vi "LJM_eAddresses Example.vi"() -> (0 "error out":errorcluster)   [LabVIEW 2020]
panel:
  in  "Write/Read":i32[](array[ring])=[1, 1, 0, 0, 0, 0] items=["Read", "Write"]
  out "Values Out":dbl[][](array[numeric]) format="%.2f"
  in  "Values In":dbl[][](array[numeric])=[[2.5], [12345.0], [0.0], [0.0], [0.0], [0.0]] format="%.2f"
  in  "NumValues":u16[](array[numeric])=[1, 1, 1, 1, 1, 1]
  in  "Types":u8[](array[numeric])=[3, 0, 0, 1, 3, 3]
  in  "Addresses":u16[](array[numeric])=[1000, 55110, 55110, 60028, 60000, 60004]
  out "Error String":string
  out "ConnectionType Out":i32
  out "DeviceType Out":i32
  in  "Identifier":string="LJM_idANY"
  in  "ConnectionType":string="LJM_ctANY"
  in  "DeviceType":string="LJM_dtANY"
  out "ErrorAddress":i32
  # "Common Registers:\nAddress, Name, Type, Read/Write\n0, AIN0, 3, RO\n2, AIN1, 3, RO\n1000, DAC0, 3, RW\n1002, DAC1, 3, RW\n2000, FIO0, 0, RW\n2001, FIO1, 0, RW\n55110, TEST_UINT16, 0, RW\n60000, PRODUCT_ID, 3, RO\n60004, FIRMWARE_VERSION, 3, RO\n60028, SERIAL_NUMBER, 1, RO\n\nTypes: 0=UINT16, 1=UINT32, 2=INT32, 3=FLOAT32"
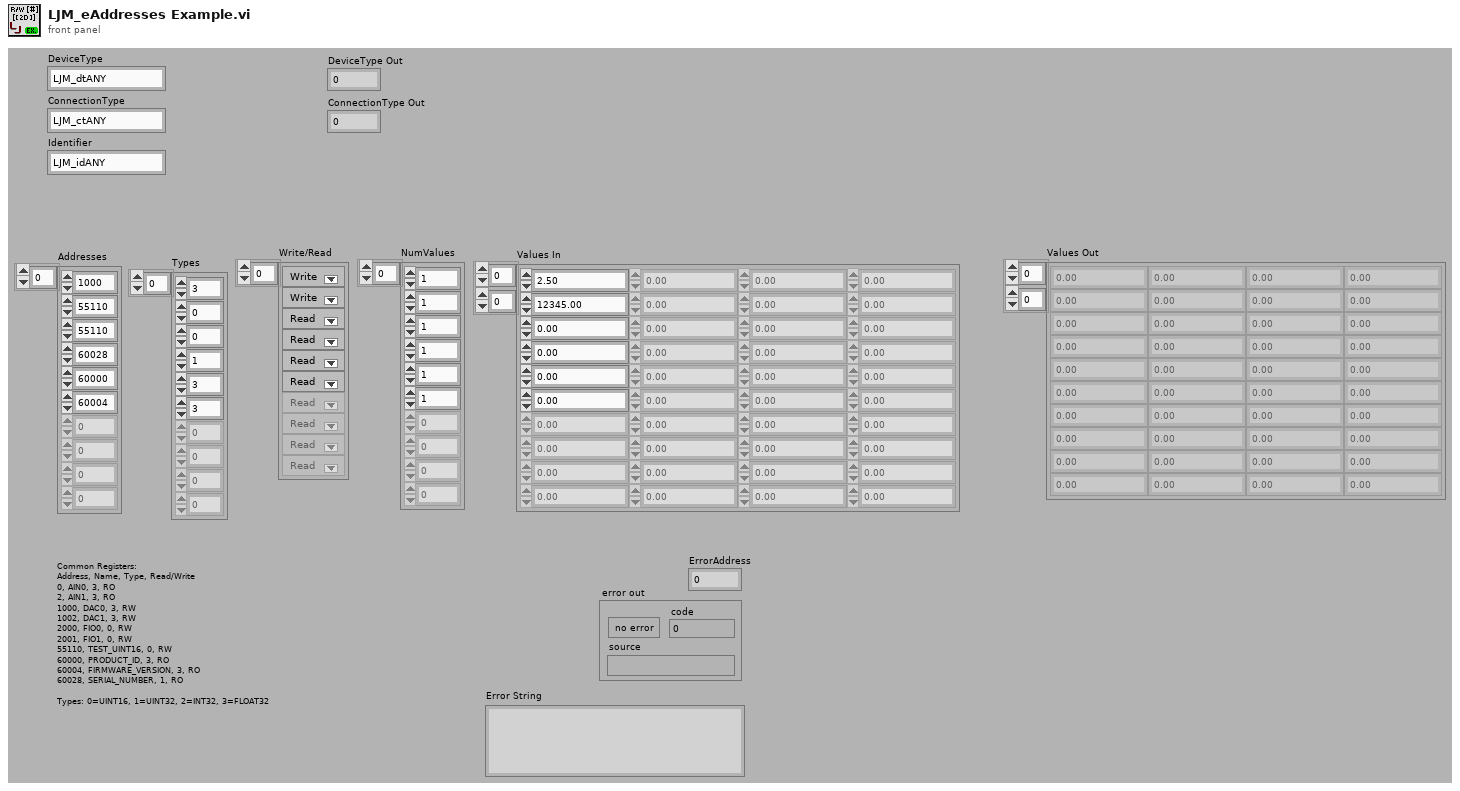
[diagram p1: front panel]
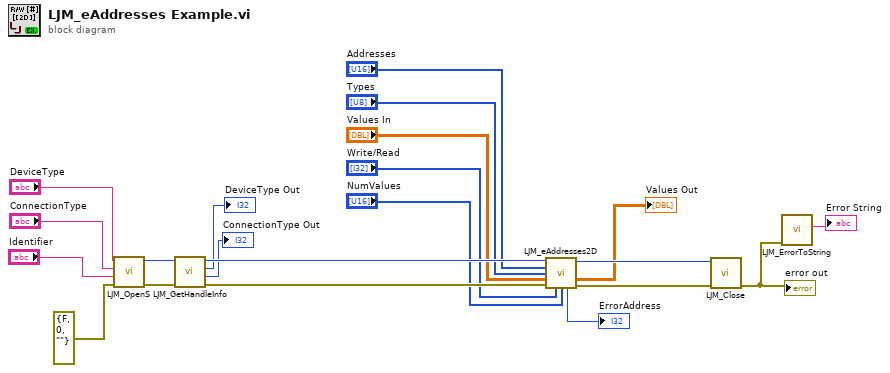
[diagram p0: block diagram]
diagram:
  n1 = call "LJM_OpenS.vi"("error in"=errorcluster {"status"=FALSE, "code"=0, "source"=""} ("error in (no error)"), "Identifier"="Identifier", "ConnectionType"="ConnectionType", "DeviceType"="DeviceType") -> ("error out"=w19:errorcluster, "Handle"=w17:i32)  [unwired: 6 in]
  n2 = call "LJM_GetHandleInfo.vi"("error in"=w19, "Handle In"=w17) -> ("error out"=w18:errorcluster, "ConnectionType"=→"ConnectionType Out":i32, "DeviceType"=→"DeviceType Out":i32, "Handle Out"=w16:i32)  [unwired: 2 in, 4 out]
  n3 = call "LJM_eAddresses2D.vi"("Handle In"=w16, "aAddresses"="Addresses", "aTypes"="Types", "aValuesIn"="Values In", "error in"=w18, "aWrites"="Write/Read", "aNumValues"="NumValues") -> ("Handle Out"=w15:i32, "aValuesOut"=→"Values Out":dbl[][], "ErrorAddress"=→"ErrorAddress":i32, "error out"=w20:errorcluster)  [unwired: 5 in]
  n4 = call "LJM_Close.vi"("error in"=w20, "Handle"=w15) -> ("error out"=w9:errorcluster)  [unwired: 9 in]
  "error out" <- w9
  n5 = call "LJM_ErrorToString.vi"("error in"=w9) -> ("String"=→"Error String":string)  [unwired: 10 in]
